vi "m1m3_getNextSample_HardpointMonitorStatus.vi"(8 "error in (no error)":errorcluster, 11 "HardpointMonitorStatus_Ctl":T1) -> (0 "error out":errorcluster, 2 "function return":i32, 3 "HardpointMonitorStatus_Ctl out":T1)   [LabVIEW 2016, in "SALLV_m1m3.lvlib"]
doc: "int m1m3_shm_getNextSample_HardpointMonitorStatusLV(m1m3_HardpointMonitorStatusLV *HardpointMonitorStatus_Ctl );"
uses:
  SALLV_m1m3.lvlib
  DataTypes/HardpointMonitorStatus.ctl
  SALLV_m1m3.so
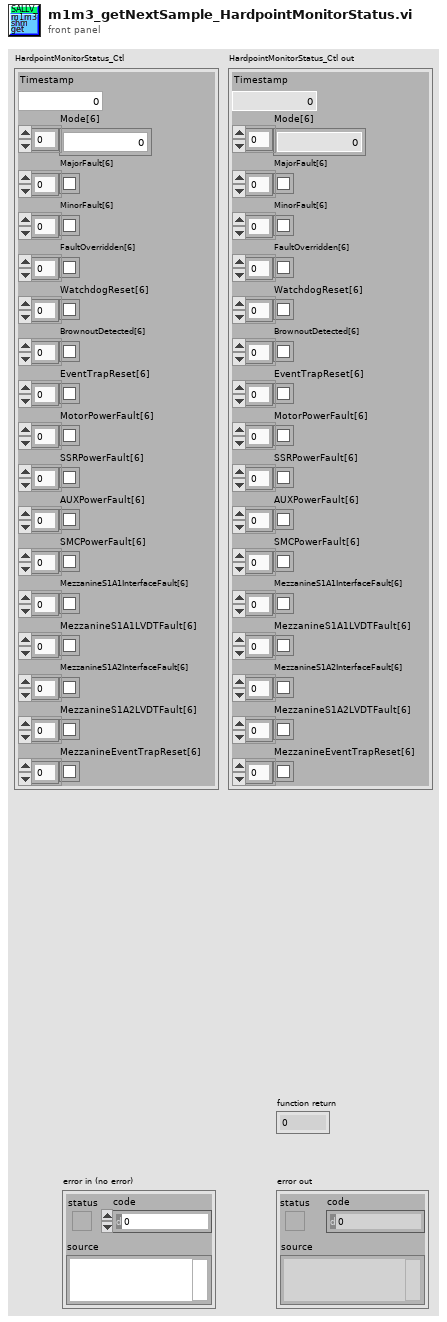
[diagram p1: front panel]
types:
  T1 = typedef "SALLV_m1m3.lvlib/HardpointMonitorStatus.ctl" = cluster{"Timestamp":dbl, "Mode[6]":u8[], "MajorFault[6]":bool[], "MinorFault[6]":bool[], "FaultOverridden[6]":bool[], "WatchdogReset[6]":bool[], "BrownoutDetected[6]":bool[], "EventTrapReset[6]":bool[], "MotorPowerFault[6]":bool[], "SSRPowerFault[6]":bool[], "AUXPowerFault[6]":bool[], "SMCPowerFault[6]":bool[], "MezzanineS1A1InterfaceFault[6]":bool[], "MezzanineS1A1LVDTFault[6]":bool[], "MezzanineS1A2InterfaceFault[6]":bool[], "MezzanineS1A2LVDTFault[6]":bool[], "MezzanineEventTrapReset[6]":bool[]}
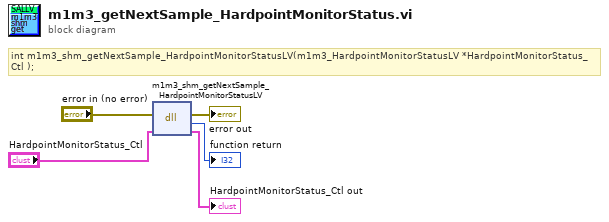
[diagram p0: block diagram]
diagram:
  # "int m1m3_shm_getNextSample_HardpointMonitorStatusLV(m1m3_HardpointMonitorStatusLV *HardpointMonitorStatus_Ctl );"
  n1 = dll-call lib="opt/CODE/SALLV_m1m3/SALLV_m1m3.*" fn="m1m3_shm_getNextSample_HardpointMonitorStatusLV"(error in="error in (no error)", "HardpointMonitorStatus_Ctl"="HardpointMonitorStatus_Ctl") -> (error out=→"error out":errorcluster, →"function return":i32, "HardpointMonitorStatus_Ctl"=→"HardpointMonitorStatus_Ctl out":T1)  [unwired: 2 in, 1 out]
